vi "CreateFile.vi"(6 "error in":errorcluster, 8 "File control":T1={"Subject ID"="", "Eye"=FALSE, "Output Path"=path "F:/MM042", "String"="", "String 2"=""}, 9 "Scan":refnum<class "Scan.lvclass">, 10 "Camera":refnum<class "Camera.lvclass">) -> (0 "error out":errorcluster, 2 "OCT filename":string, 3 "refnum out":refnum<file>)   [LabVIEW 2017]
uses:
  classes/HardwareObjects/Camera/Camera.lvclass
  classes/Scans/Scan.lvclass
  classes/HardwareObjects/Camera/Camera.lvclass/Camera.ctl
  classes/Scans/Scan.lvclass/Scan.ctl
  classes/Scans/Read A scans.vi
  classes/Scans/Read B scans.vi
  classes/Scans/Read Bidirectional.vi
  classes/Scans/Read C scans.vi
  classes/Scans/Read Repeat B scans.vi
  classes/Scans/Read Scan Angle (degrees).vi
  classes/Scans/Read Scan Pattern.vi
  classes/Scans/Read X FOV (degrees).vi
  classes/Scans/Read X offset (degrees).vi
  classes/Scans/Read Y offset (degrees).vi
  classes/HardwareObjects/Camera/Read Bit Depth.vi
  classes/HardwareObjects/Camera/Read Camera Dimensions.vi
  classes/HardwareObjects/Camera/Read Data Representation.vi
  classes/HardwareObjects/Camera/Read Duty Cycle.vi
  classes/HardwareObjects/Camera/Read Max Frequency (kHz).vi
  classes/HardwareObjects/Camera/Read Return Time (us).vi
panel:
  out "Eye indicator":string
  out "Header filename":string
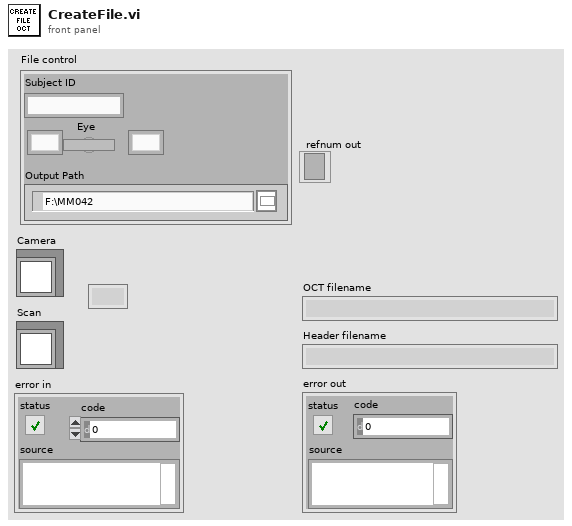
[diagram p1: front panel]
types:
  T1 = cluster{"Subject ID":string, "Eye":bool, "Output Path":path, "String":string, "String 2":string}
  T2 = enum16{"big-endian, network order", "native, host order", "little-endian"}
  T3 = enum16{"open", "replace", "create", "open or create", "replace or create", "replace or create with confirmation"}
  T4 = cluster{"string":string, "string":string, "string":string, "Scan Angle 2D":dbl, "string":string, "X offset (degrees)":dbl, "string":string, "Y offset (degrees)":dbl, "string":string, "Scan Angle (degrees)":dbl, "string":string, "X FOV (degrees)":dbl, "string":string, "A scans":dbl, "string":string, "B scans":dbl}
  T5 = cluster{"string":string, dbl, "string":string, "Return Time (µs)":sgl, "string":string, "Max Frequency (kHz)":sgl, "string":string, dbl, "string":string, "Duty Cycle":sgl, "string":string, "Max Frequency (kHz)":sgl}
  T6 = cluster{cluster{"string":string, "string":string, "string":string, "Scan Angle 2D":dbl, "string":string, "X offset (degrees)":dbl, "string":string, "Y offset (degrees)":dbl, "string":string, "Scan Angle (degrees)":dbl, "string":string, "X FOV (degrees)":dbl, "string":string, "A scans":dbl, "string":string, "B scans":dbl}, cluster{"string":string, dbl, "string":string, "Return Time (µs)":sgl, "string":string, "Max Frequency (kHz)":sgl, "string":string, dbl, "string":string, "Duty Cycle":sgl, "string":string, "Max Frequency (kHz)":sgl}, cluster{"string":string, "Repeat B scans":dbl}, "string":string, "string":string}
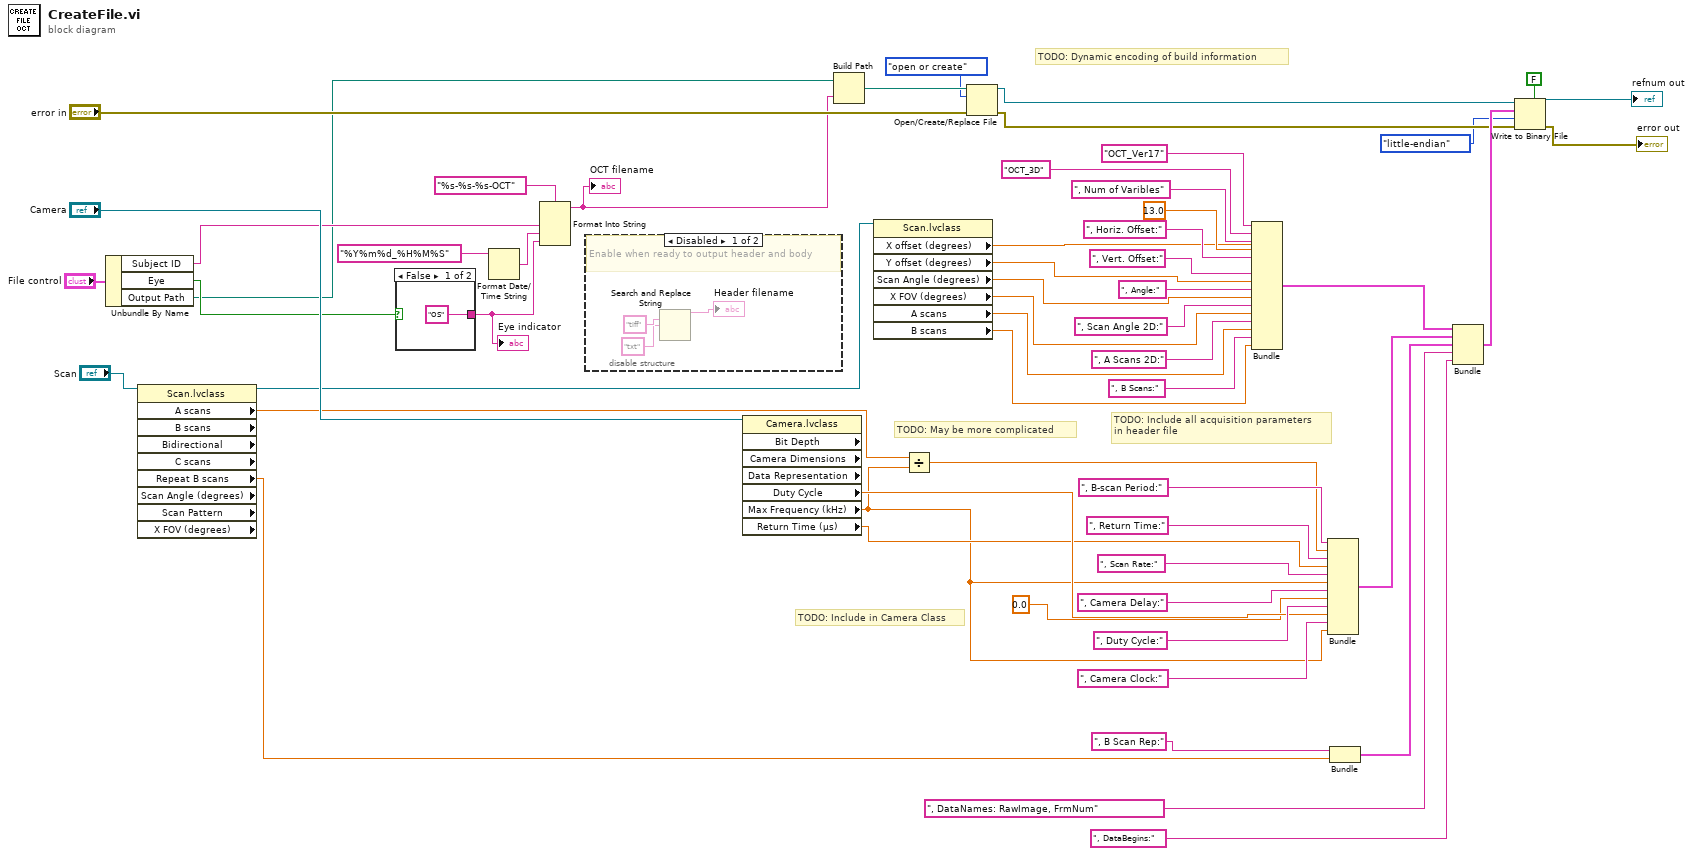
[diagram p0: block diagram]
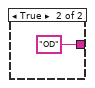
[diagram p3: hidden frame]
diagram:
  # "TODO: Include all acquisition parameters\nin header file"
  # "TODO: May be more complicated"
  # "TODO: Include in Camera Class"
  # "TODO: Dynamic encoding of build information"
  n1 = Unbundle By Name("File control") -> ("Subject ID"=w2:string, "Eye"=w3:bool, "Output Path"=w1:path)
  n2 = property class="Scan.lvclass" props=["A scans", "B scans", "Bidirectional", "C scans", "Repeat B scans", "Scan Angle (degrees)", "Scan Pattern", "X FOV (degrees)"](reference="Scan") -> (reference out=w17:refnum<class "Scan.lvclass">, "A scans"=w18:dbl, "Repeat B scans"=w22:dbl)  [unwired: 1 in, 7 out]
  n3 = case shown="False" w3 {
    tunnel: ["OS" "OD"] -> w7
    frame False {
    }
    frame True {
    }
  }
  "Eye indicator" <- w7
  n4 = Format Date/Time String(time format string (%c)="%Y%m%d_%H%M%S") -> (date/time string=w9:string)  [unwired: 2 in]
  n5 = Format Into String(format string="%s-%s-%s-OCT", w2, w9, w7) -> (resulting string=w6:string)  [unwired: 2 in, 1 out]
  "OCT filename" <- w6
  n6 = disable-structure shown="Disabled" {
    frame Disabled {
      # "Enable when ready to output header and body"
      n7 = Search and Replace String(search string="tiff", replace string="txt" ("replace string (\"\")")) -> (result string=→"Header filename":string)  [unwired: 6 in, 3 out]
    }
    frame Enabled {
    }
  }
  n8 = property class="Camera.lvclass" props=["Bit Depth", "Camera Dimensions", "Data Representation", "Duty Cycle", "Max Frequency (kHz)", "Return Time (µs)"](reference="Camera") -> ("Duty Cycle"=w24:sgl, "Max Frequency (kHz)"=w21:sgl, "Return Time (µs)"=w23:sgl)  [unwired: 1 in, 5 out]
  n9 = Build Path(base path=w1, name or relative path=w6) -> (appended path=w57:path)
  n10 = property class="Scan.lvclass"(reference=w17) -> ("X offset (degrees)"=w16:dbl, "Y offset (degrees)"=w15:dbl, "Scan Angle (degrees)"=w14:dbl, "X FOV (degrees)"=w13:dbl, "A scans"=w12:dbl, "B scans"=w11:dbl)  [unwired: 1 in, 2 out]
  n11 = Divide(x=w18, y=w21) -> (x/y=w20:dbl)
  n12 = Open/Create/Replace File(file path (use dialog)=w57, error in="error in", operation (0:open)=T3."open or create") -> (refnum out=w40:refnum<file>, error out=w39:errorcluster)  [unwired: 3 in, 1 out]
  n13 = Bundle("string"="OCT_Ver17", "string"="OCT_3D", "string"=", Num of Varibles", "Scan Angle 2D"=13.0, "string"=", Horiz. Offset:", "X offset (degrees)"=w16, "string"=", Vert. Offset:", "Y offset (degrees)"=w15, "string"=", Angle:", "Scan Angle (degrees)"=w14, "string"=", Scan Angle 2D:", "X FOV (degrees)"=w13, "string"=", A Scans 2D:", "A scans"=w12, "string"=", B Scans:", "B scans"=w11) -> (w43:T4)  [unwired: 1 in]
  n14 = Bundle("string"=", B-scan Period:", w20, "string"=", Return Time:", "Return Time (µs)"=w23, "string"=", Scan Rate:", "Max Frequency (kHz)"=w21, "string"=", Camera Delay:", 0.0, "string"=", Duty Cycle:", "Duty Cycle"=w24, "string"=", Camera Clock:", "Max Frequency (kHz)"=w21) -> (w42:T5)  [unwired: 1 in]
  n15 = Bundle("string"=", B Scan Rep:", "Repeat B scans"=w22) -> (w30:cluster{"string":string, "Repeat B scans":dbl})  [unwired: 1 in]
  n16 = Bundle(w43, w42, w30, "string"=", DataNames: RawImage, FrmNum", "string"=", DataBegins:") -> (w41:T6)  [unwired: 1 in]
  n17 = Write to Binary File(file (use dialog)=w40, data=w41, error in=w39, 5:FALSE ("prepend array or string size? (T)"), 9:T2."little-endian" ("byte order (0:big-endian, network order)")) -> (refnum out=→"refnum out":refnum<file>, error out=→"error out":errorcluster)  [unwired: 1 in, 1 out]
